vi "Log.vi"(8 "error in":errorcluster, 10 "LogIn":string, 11 "Info":T1) -> ()   [LabVIEW 2018]
uses:
  <userlib>/_MGI/File/MGI Create Directory Chain Behavior Enum.ctl
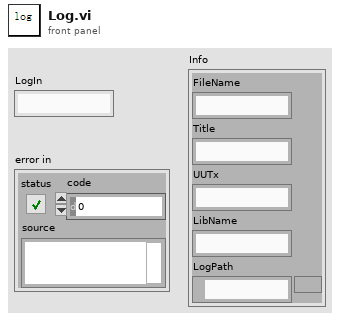
[diagram p1: front panel]
types:
  T1 = cluster{"FileName":string, "Title":string, "UUTx":string, "LibName":string, "LogPath":path}
  T2 = typedef "MGI Create Directory Chain Behavior Enum.ctl" = enum16{"Auto Detect", "Path Contains a File", "Path Does Not Contain a File"}
  T3 = enum16{"open", "replace", "create", "open or create", "replace or create", "replace or create with confirmation"}
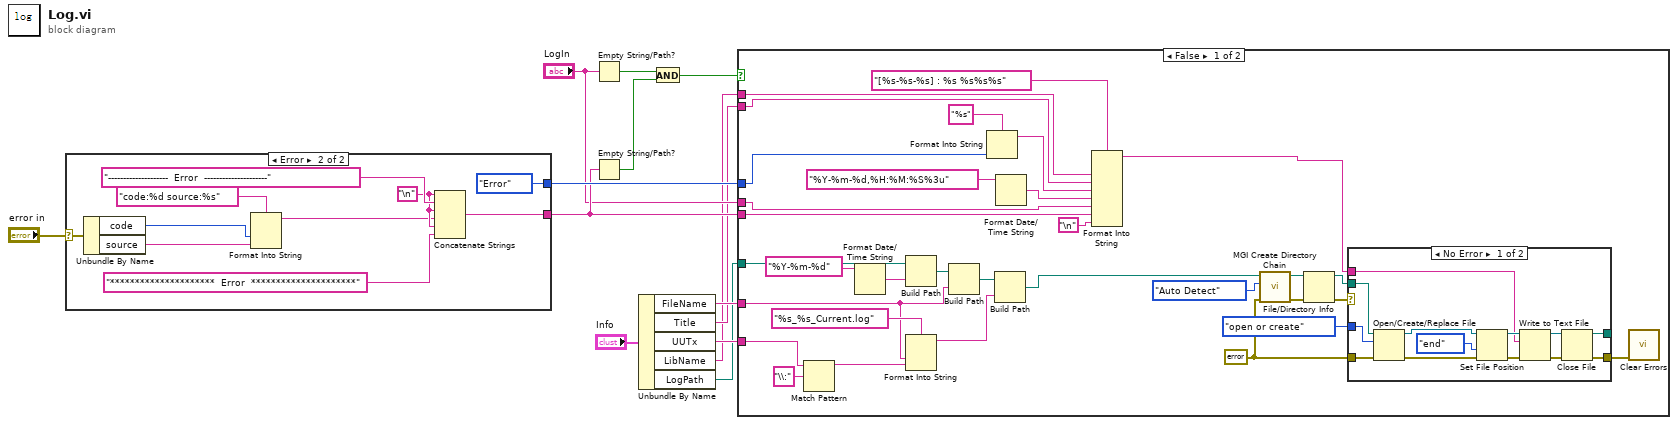
[diagram p0: block diagram]
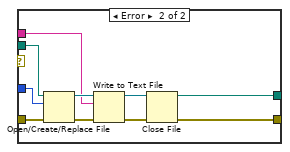
[diagram p2: hidden frame]
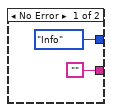
[diagram p4: hidden frame]
diagram:
  n1 = case shown="Error" "error in" {
    selector: "error in" -> [_ w24]
    tunnel: ["" w18] -> w11
    tunnel: [enum16{"Info", "Error", "Debug"}."Info" ("LogType") enum16{"Info", "Error", "Debug"}."Error" ("LogType")] -> w12
    frame No Error {
    }
    frame Error {
      w23 = "\n"
      n2 = Unbundle By Name(w24) -> ("code"=w21:i32, "source"=w20:string)
      n3 = Format Into String(format string="code:%d source:%s", w21, w20) -> (resulting string=w19:string)  [unwired: 2 in, 1 out]
      n4 = Concatenate Strings(w23, "--------------------  Error  ---------------------" ("string"), w23, w19, w23, "*********************  Error  *********************" ("string")) -> (w18:string)
    }
  }
  n5 = Empty String/Path?(string/path="LogIn") -> (empty?=w9:bool)
  n6 = Empty String/Path?(string/path=w11) -> (empty?=w8:bool)
  n7 = Unbundle By Name("Info") -> ("FileName"=w5:string, "Title"=w4:string, "UUTx"=w3:string, "LibName"=w2:string, "LogPath"=w1:path)
  n8 = And(x=w9, y=w8) -> (x .and. y?=w7:bool)
  n9 = case shown="False" w7 {
    tunnel: w1 -> [w37 _]
    tunnel: w12 -> [w33 _]
    tunnel: w11 -> [w31 _]
    tunnel: "LogIn" -> [w32 _]
    tunnel: w5 -> [w36 _]
    tunnel: w2 -> [w35 _]
    tunnel: w4 -> [w34 _]
    tunnel: w3 -> [w28 _]
    frame False {
      w48 = errorcluster {"status"=FALSE, "code"=0, "source"=""} ("error out")
      n10 = Match Pattern(string=w28, regular expression="\\:") -> (before substring=w26:string)  [unwired: 1 in, 3 out]
      n11 = Format Date/Time String(time format string (%c)="%Y-%m-%d") -> (date/time string=w50:string)  [unwired: 2 in]
      n12 = Build Path(base path=w37, name or relative path=w50) -> (appended path=w51:path)
      n13 = Format Into String(format string="%s_%s_Current.log", w36, w26) -> (resulting string=w43:string)  [unwired: 2 in, 1 out]
      n14 = Build Path(base path=w51, name or relative path=w36) -> (appended path=w46:path)
      n15 = Format Into String(format string="%s", w33) -> (resulting string=w39:string)  [unwired: 2 in, 1 out]
      n16 = Build Path(base path=w46, name or relative path=w43) -> (appended path=w29:path)
      n17 = Format Date/Time String(time format string (%c)="%Y-%m-%d,%H:%M:%S%3u") -> (date/time string=w41:string)  [unwired: 2 in]
      n18 = Format Into String(format string="[%s-%s-%s] : %s %s%s%s", w35, w34, w39, w41, w32, w31, "\n") -> (resulting string=w45:string)  [unwired: 2 in, 1 out]
      n19 = call <userlib>:"MGI Create Directory Chain.vi"("Error In"=w48, "File Presence (Auto Detect)"=MGI_Create_Directory_Chain_Behavior_Enum."Auto Detect", "Path"=w29) -> ("Error Out"=w56:errorcluster, "Duplicate Path"=w57:path)  [unwired: 7 in]
      n20 = File/Directory Info(path=w57, error in=w56) -> (path out=w54:path, error out=w55:errorcluster)  [unwired: 5 out]
      n21 = case shown="No Error" w55 {
        tunnel: w54 -> [w70 w73]
        tunnel: T3."open or create" ("operation (0:open)") -> [w69 w71]
        tunnel: w48 -> [w68 w72]
        tunnel: w45 -> [w62 w74]
        tunnel: [w59 w78] -> _
        tunnel: [w58 w77] -> w47
        frame No Error {
          n22 = Open/Create/Replace File(file path (use dialog)=w70, error in=w68, operation (0:open)=w69) -> (refnum out=w67:refnum<file>, error out=w66:errorcluster)  [unwired: 3 in, 1 out]
          n23 = Set File Position(refnum=w67, from (0:start)=enum16{"start", "end", "current"}."end", error in=w66) -> (refnum out=w64:refnum<file>, error out=w63:errorcluster)  [unwired: 1 in]
          n24 = Write to Text File(file (use dialog)=w64, text=w62, error in=w63) -> (refnum out=w60:refnum<file>, error out=w61:errorcluster)  [unwired: 1 in, 1 out]
          n25 = Close File(refnum=w60, error in=w61) -> (path=w59:path, error out=w58:errorcluster)
        }
        frame Error {
          n26 = Open/Create/Replace File(file path (use dialog)=w73, error in=w72, operation (0:open)=w71) -> (refnum out=w76:refnum<file>, error out=w75:errorcluster)  [unwired: 3 in, 1 out]
          n27 = Write to Text File(file (use dialog)=w76, text=w74, error in=w75) -> (refnum out=w79:refnum<file>, error out=w80:errorcluster)  [unwired: 1 in, 1 out]
          n28 = Close File(refnum=w79, error in=w80) -> (path=w78:path, error out=w77:errorcluster)
        }
      }
      n29 = call <vilib>:"Clear Errors.vi"("error in (no error)"=w47) -> ()  [unwired: 5 in, 2 out]
    }
    frame True {
    }
  }
